vi "OrderFreqAmpl.vi"(1 "Size":i32=6, 2 "Amplitude":dbl[](array[numeric]), 3 "Frequencies":dbl[](array[numeric])) -> (0 "appended array":dbl[][](array[numeric]))   [LabVIEW 2016]
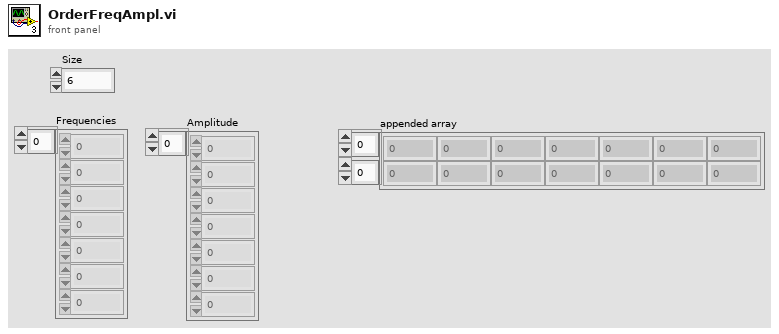
[diagram p1: front panel]
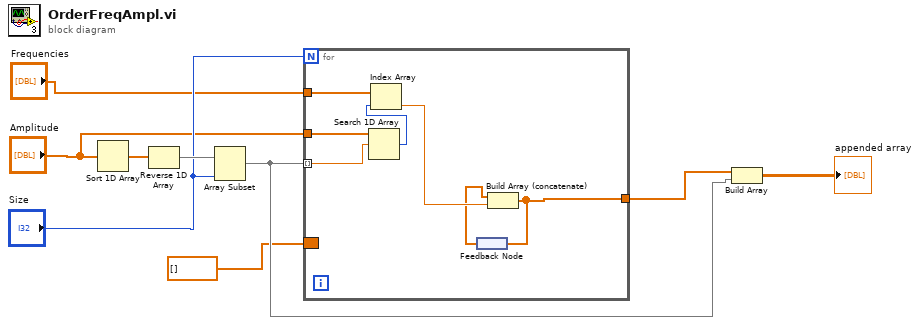
[diagram p0: block diagram]
diagram:
  n1 = Sort 1D Array(array="Amplitude") -> (sorted array=w9:dbl[])
  n2 = Reverse 1D Array(array=w9) -> (reversed array=w8:dbl[])
  n3 = Array Subset(array=w8, length="Size") -> (w2:dbl[])  [unwired: 1 in]
  n4 = for {
    N: "Size" -> [_]
    tunnel: "Amplitude" -> [w16]
    tunnel: w2 -> [w15] mode=indexing
    tunnel: "Frequencies" -> [w13]
    tunnel: [w10] -> w5
    border: dbl[] [] -> [_]
    n5 = Search 1D Array(1D array=w16, element=w15) -> (index of element=w14:i32)  [unwired: 1 in]
    n6 = Index Array(array=w13, index=w14) -> (element=w12:dbl)
    n7 = feedback #1() -> (w11:dbl[])
    n8 = Build Array (concatenate)(w11, w12) -> (w10:dbl[])
    n9 = feedback-in #1(w10) -> ()
  }
  n10 = Build Array(w5, w2) -> (→"appended array":dbl[][])
